vi "ma_SML Exponential Weighting (real input).vi"(2 "reset?":bool, 3 "average size":dbl, 4 "x":dbl[](array[numeric]) format="%.2f") -> (0 "averaged sofar":dbl, 1 "y":dbl[](array[numeric]) format="%.2f")   [LabVIEW 2020, in "NI_MAPro.lvlib"]
uses:
  NI_MAPro.lvlib
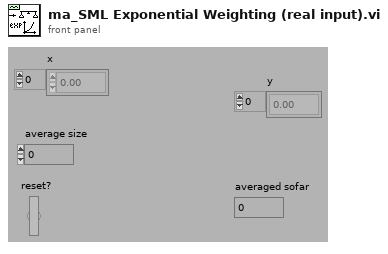
[diagram p1: front panel]
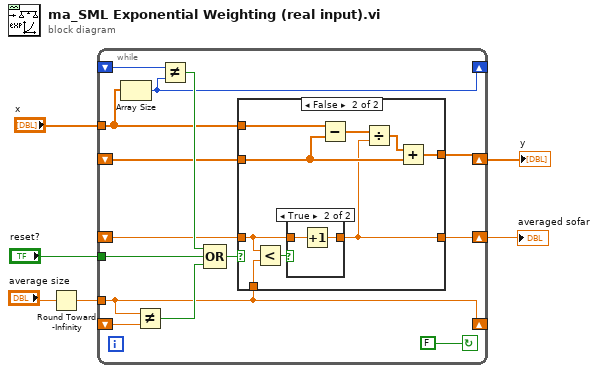
[diagram p0: block diagram]
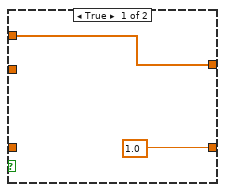
[diagram p2: hidden frame]
diagram:
  n1 = Round Toward -Infinity(1:"average size") -> (0:w3:dbl)
  n2 = while {
    tunnel: "x" -> [w11]
    shift-left: _ -> [w18]
    shift-right: [w17] -> _
    tunnel: w3 -> [w7]
    shift-left: _ -> [w16]
    shift-right: [w7] -> _
    shift-left: _ -> [w12]
    shift-right: [w13] -> w4
    shift-left: _ -> [w10]
    shift-right: [w9] -> w1
    tunnel: "reset?" -> [w20]
    stop <- FALSE continue-if-true
    n3 = Array Size(array=w11) -> (size(s)=w17:i32)
    n4 = Not Equal?(x=w7, y=w16) -> (x != y?=w15:bool)
    n5 = Not Equal?(x=w18, y=w17) -> (x != y?=w19:bool)
    n6 = Compound Arithmetic op=OR(w19, w20, w15) -> (w14:bool)
    n7 = case shown="False" w14 {
      tunnel: w11 -> [w21 w28]
      tunnel: [1.0 w23] -> w13
      tunnel: w12 -> [_ w29]
      tunnel: w7 -> [_ w31]
      tunnel: w10 -> [_ w24]
      tunnel: [w21 w26] -> w9
      frame True {
      }
      frame False {
        n8 = Less?(x=w29, y=w31) -> (x < y?=w30:bool)
        n9 = case shown="True" w30 {
          tunnel: w29 -> [w32 w34]
          tunnel: [w32 w33] -> w23
          frame False {
          }
          frame True {
            n10 = Increment(x=w34) -> (x+1=w33:dbl)
          }
        }
        n11 = Subtract(x=w28, y=w24) -> (x-y=w27:dbl[])
        n12 = Divide(x=w27, y=w23) -> (x/y=w25:dbl[])
        n13 = Add(x=w25, y=w24) -> (x+y=w26:dbl[])
      }
    }
  }
  "averaged sofar" <- w4
  "y" <- w1
